vi "Table Copy To Clipboard.vi"(2 "cut (False)":bool, 3 "signaling change (False)":bool, 4 "table ref":refnum<vi>) -> (0 "all data":string[][](array[string]), 1 "copied data":string[][](array[string]))   [LabVIEW 2020]
doc: "Copies table range to clipboard."
panel:
  out "spreadsheet string":string
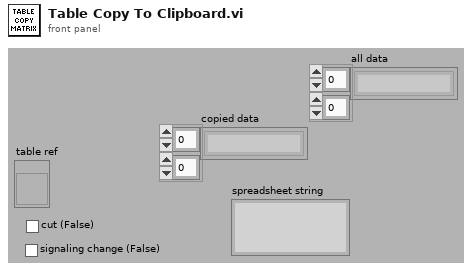
[diagram p1: front panel]
types:
  T1 = typedef "LVRowAndColumnTypeDef.ctl" = cluster{"Row":i32, "Column":i32}
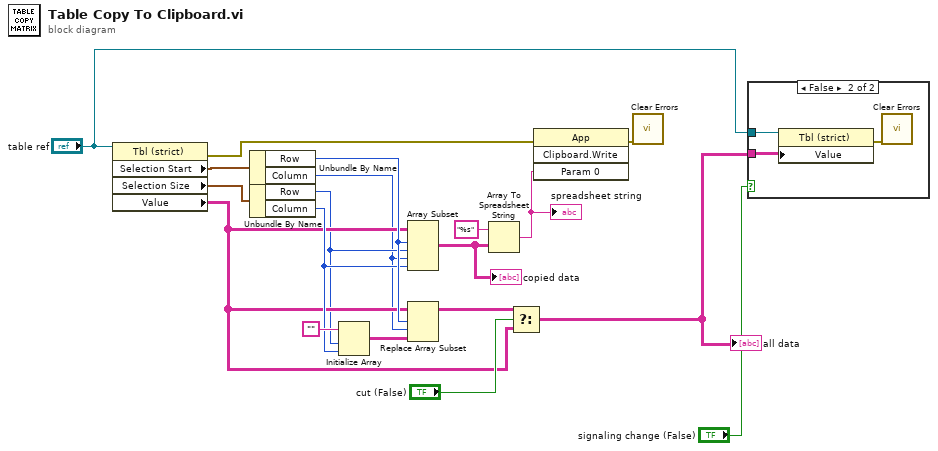
[diagram p0: block diagram]
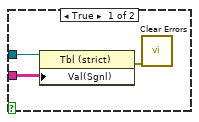
[diagram p2: hidden frame]
diagram:
  n1 = property on="Property Node" class="Tbl (strict)"(reference="table ref") -> (error out=w14:errorcluster, "Selection Start"=w19:T1, "Selection Size"=w16:T1, "Value"=w4:string[][])  [unwired: 1 in, 1 out]
  n2 = Unbundle By Name(w19) -> ("Row"=w10:i32, "Column"=w1:i32)
  n3 = Unbundle By Name(w16) -> ("Row"=w2:i32, "Column"=w8:i32)
  n4 = Initialize Array("", w2, w8) -> (w7:string[][])
  n5 = Array Subset(array=w4, index (row)=w10, length (row)=w2, index (col)=w1, length (col)=w8) -> (w11:string[][])
  "copied data" <- w11
  n6 = Replace Array Subset(array=w4, new element=w7, index (row)=w10, index (col)=w1) -> (w5:string[][])
  n7 = Array To Spreadsheet String(array=w11, 3:"%s" ("format string")) -> (spreadsheet string=w13:string)  [unwired: 1 in]
  "spreadsheet string" <- w13
  n8 = Select(t=w5, s="cut (False)", f=w4) -> (s? t:f=w3:string[][])
  "all data" <- w3
  n9 = invoke class="App" method="Clipboard.Write"(error in=w14, "Param 0"=w13) -> (error out=w12:errorcluster)  [unwired: 2 in, 3 out]
  n10 = call <vilib>:"Clear Errors.vi"("error in (no error)"=w12) -> ()  [unwired: 5 in, 2 out]
  n11 = case shown="False" "signaling change (False)" {
    tunnel: w3 -> [w22 w25]
    tunnel: "table ref" -> [w21 w24]
    frame True {
      n12 = property on="Property Node" class="Tbl (strict)"(reference=w21, "Val(Sgnl)"=w22) -> (error out=w20:errorcluster)  [unwired: 1 in, 1 out]
      n13 = call <vilib>:"Clear Errors.vi"("error in (no error)"=w20) -> ()  [unwired: 5 in, 2 out]
    }
    frame False {
      n14 = property on="Property Node" class="Tbl (strict)"(reference=w24, "Value"=w25) -> (error out=w23:errorcluster)  [unwired: 1 in, 1 out]
      n15 = call <vilib>:"Clear Errors.vi"("error in (no error)"=w23) -> ()  [unwired: 5 in, 2 out]
    }
  }
